vi "题目2.vi"() -> ()   [LabVIEW 2017]
panel:
  out "数值 2":dbl
  out "数值":dbl
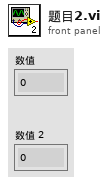
[diagram p1: front panel]
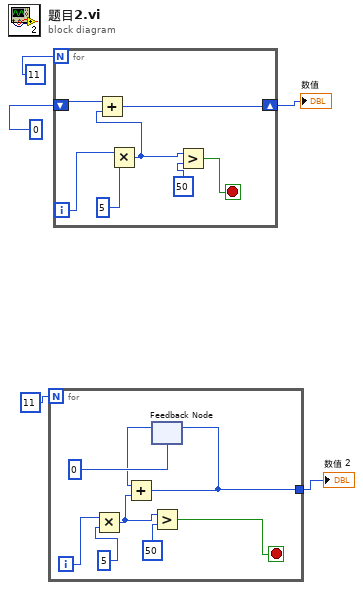
[diagram p0: block diagram]
diagram:
  n1 = for {
    N: 11 -> [_]
    tunnel: [w7] -> w2
    i -> [w13]
    stop <- w10 stop-if-true
    n2 = Multiply(x=w13, y=5) -> (x*y=w6:i32)
    n3 = feedback #1(0) -> (w8:i32)
    n4 = Add(x=w8, y=w6) -> (x+y=w7:i32)
    n5 = feedback-in #1(w7) -> ()
    n6 = Greater?(x=w6, y=50) -> (0:w10:bool)
  }
  "数值 2" <- w2
  n7 = for {
    N: 11 -> [_]
    shift-right: [w17] -> w3
    shift-left: 0 -> [w18]
    i -> [w19]
    stop <- w14 stop-if-true
    n8 = Multiply(x=w19, y=5) -> (x*y=w16:i32)
    n9 = Add(x=w18, y=w16) -> (x+y=w17:i32)
    n10 = Greater?(x=w16, y=50) -> (0:w14:bool)
  }
  "数值" <- w3
